vi "setVipBuildNumber.vi"() -> ()   [LabVIEW 2014, in "lv-cli-steps.lvlib"]
uses:
  lv-cli-steps.lvlib
  <vilib>/JKI/VIPM API/command-line/support/VI Package Build Spec Data Cluster_vipm_api.ctl
  <vilib>/JKI/VIPM API/command-line/support/Version Info Cluster_vipm_api.ctl
  <vilib>/Utility/error.llb/DialogType.ctl
  <vilib>/JKI/VIPM API/VIPM API_vipm_api.lvlib
  <vilib>/Wiresmith Technology/LabVIEW CLI/CLI Class/CLI.lvclass
panel:
  out "Next build number":u32
  out "error out":errorcluster
  out "VI Package Build Spec Data":T1
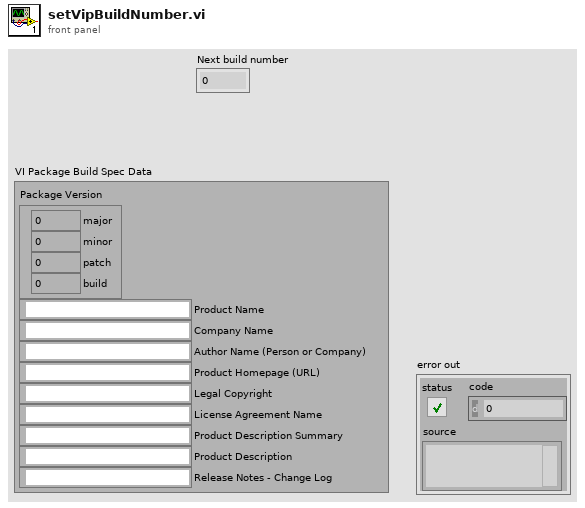
[diagram p1: front panel]
types:
  T1 = typedef "VIPM API_vipm_api.lvlib/VI Package Build Spec Data Cluster_vipm_api.ctl" = cluster{"Package Version":T2, "Product Name":string, "Company Name":string, "Author Name (Person or Company)":string, "Product Homepage (URL)":string, "Legal Copyright":string, "License Agreement Name":string, "Product Description Summary":string, "Product Description":string, "Release Notes - Change Log":string}
  T2 = typedef "VIPM API_vipm_api.lvlib/Version Info Cluster_vipm_api.ctl" = cluster{"major":u32, "minor":u32, "patch":u32, "build":u32}
  T3 = typedef "VIPM API_vipm_api.lvlib/Repository Contents Cluster_vipm_api.ctl" = cluster{"Package Name":string, "Version":string, "Display Name":string, "Release Date":string, "Deprecated":bool}
  T4 = typedef "DialogType.ctl" = u16
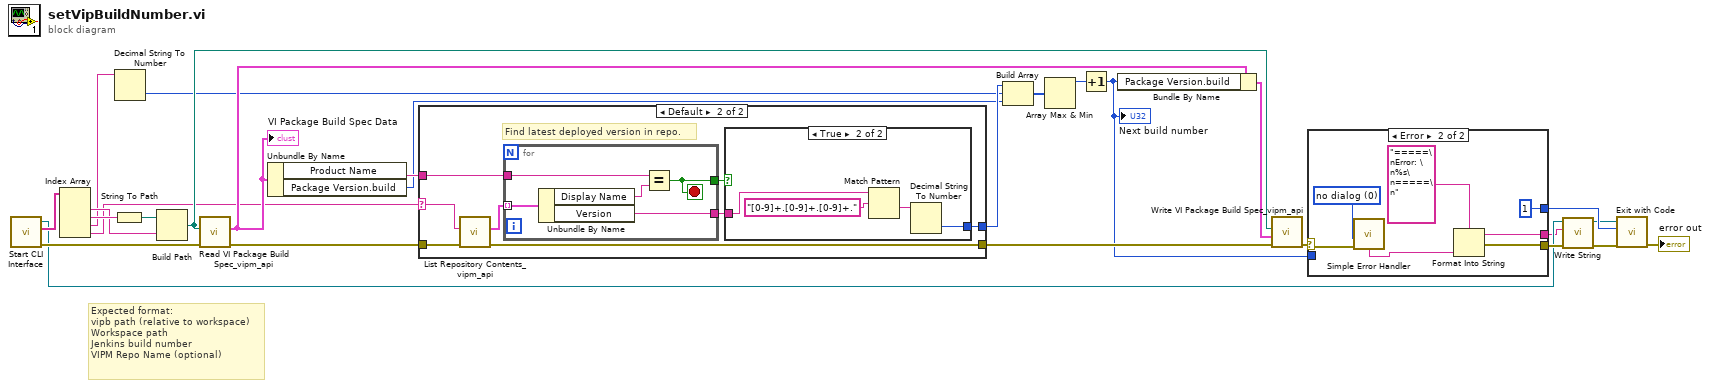
[diagram p0: block diagram]
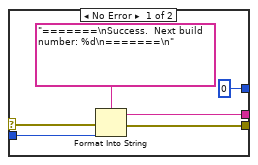
[diagram p2: hidden frame]
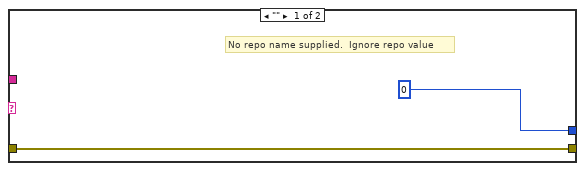
[diagram p3: hidden frame]
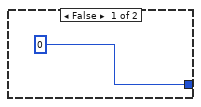
[diagram p4: hidden frame]
diagram:
  # "Expected format:\nvipb path (relative to workspace)\nWorkspace path\nJenkins build number\nVIPM Repo Name (optional)"
  n1 = call <vilib>:"Start CLI Interface.vi"() -> ("error out"=w18:errorcluster, "Custom Parameters"=w16:string[], "CLI out"=w3:refnum<class "CLI.lvclass">)  [unwired: 9 in]
  n2 = Index Array(array=w16) -> (element #1=w13:string, element #2=w15:string, element #3=w12:string, element #4=w10:string)  [unwired: 4 in]
  n3 = String To Path(string=w15) -> (path=w14:path)
  n4 = Decimal String To Number(string=w12) -> (number=w11:i32)  [unwired: 2 in, 1 out]
  n5 = Build Path(base path=w14, name or relative path=w13) -> (appended path=w17:path)
  n6 = call <vilib>:"Read VI Package Build Spec_vipm_api.vi"("error in (no error)"=w18, "Path to VIPB File"=w17) -> ("error out"=w23:errorcluster, "VI Package Build Spec Data"=w22:T1)  [unwired: 8 in]
  "VI Package Build Spec Data" <- w22
  n7 = Unbundle By Name(w22) -> ("Product Name"=w21:string, "Package Version.build"=w20:u32)
  n8 = case shown="Default" w10 {
    selector: w10 -> [_ w30]
    tunnel: [0 w35] -> w27
    tunnel: [w28 w34] -> w7
    tunnel: w23 -> [w28 w33]
    tunnel: w21 -> [_ w31]
    frame "" {
      # "No repo name supplied.  Ignore repo value"
    }
    frame Default {
      # "Find latest deployed version in repo."
      n9 = call <vilib>:"List Repository Contents_vipm_api.vi"("error in (no error)"=w33, "Repository Name"=w30) -> ("error out"=w34:errorcluster, "Repository Contents []"=w37:T3[])  [unwired: 8 in]
      n10 = for {
        tunnel: w37 -> [w47] mode=indexing
        tunnel: [w45] -> w36
        tunnel: [w44] -> w32
        tunnel: w31 -> [w43]
        stop <- w44 stop-if-true
        n11 = Unbundle By Name(w47) -> ("Display Name"=w46:string, "Version"=w45:string)
        n12 = Equal?(x=w43, y=w46) -> (x = y?=w44:bool)
      }
      n13 = case shown="True" w32 {
        tunnel: w36 -> [_ w42]
        tunnel: [0 w39] -> w35
        frame False {
        }
        frame True {
          n14 = Match Pattern(string=w42, regular expression="[0-9]+.[0-9]+.[0-9]+.") -> (after substring=w40:string)  [unwired: 1 in, 3 out]
          n15 = Decimal String To Number(string=w40) -> (number=w39:i32)  [unwired: 2 in, 1 out]
        }
      }
    }
  }
  n16 = Build Array(w27, w11, w20) -> (w26:u32[])
  n17 = Array Max & Min(array=w26) -> (max value=w25:u32)  [unwired: 3 out]
  n18 = Increment(x=w25) -> (x+1=w6:u32)
  "Next build number" <- w6
  n19 = Bundle By Name(cluster=w22, "Package Version.build"=w6) -> (w24:T1)
  n20 = call <vilib>:"Write VI Package Build Spec_vipm_api.vi"("error in (no error)"=w7, "VI Package Build Spec Data"=w24, "Path to VIPB File"=w17) -> ("error out"=w9:errorcluster)  [unwired: 8 in]
  n21 = case shown="Error" w9 {
    selector: w9 -> [w51 w57]
    tunnel: [0 ("Exit Code (0)") 1 ("Exit Code (0)")] -> w8
    tunnel: w6 -> [w50 _]
    tunnel: [w49 w59] -> w4
    tunnel: [w48 w58] -> w2
    frame No Error {
      n22 = Format Into String(format string="=======\nSuccess.  Next build number: %d\n=======\n", error in=w51, w50) -> (resulting string=w48:string, error out=w49:errorcluster)  [unwired: 1 in]
    }
    frame Error {
      w54 = T4 0 items=["no dialog", "OK message", "continue or stop message", "OK message + warnings", "continue/stop + warnings"] ("type of dialog (OK msg:1)")
      n23 = call <vilib>:"Simple Error Handler.vi"("type of dialog (OK msg:1)"=w54, "error in (no error)"=w57) -> ("message"=w55:string)  [unwired: 3 in, 4 out]
      n24 = Format Into String(format string="=====\nError: \n%s\n=====\n", w55) -> (resulting string=w58:string, error out=w59:errorcluster)  [unwired: 2 in]
    }
  }
  n25 = call <vilib>:"Write String.vi"("error in (no error)"=w4, "Text to Write"=w2, "CLI in"=w3) -> ("error out"=w5:errorcluster, "CLI out"=w1:refnum<class "CLI.lvclass">)  [unwired: 7 in]
  n26 = call <vilib>:"Exit with Code.vi"("error in (no error)"=w5, "Exit Code (0)"=w8, "CLI in"=w1) -> ("error out"=→"error out":errorcluster)  [unwired: 8 in]
